vi "MergeROIs.vi"(9 "ROI 2":T1(array[cluster]), 11 "ROI 1":T1(array[cluster])) -> (3 "Merged ROI":T1(array[cluster]))   [LabVIEW 2014]
panel:
  in  "ROI":T2
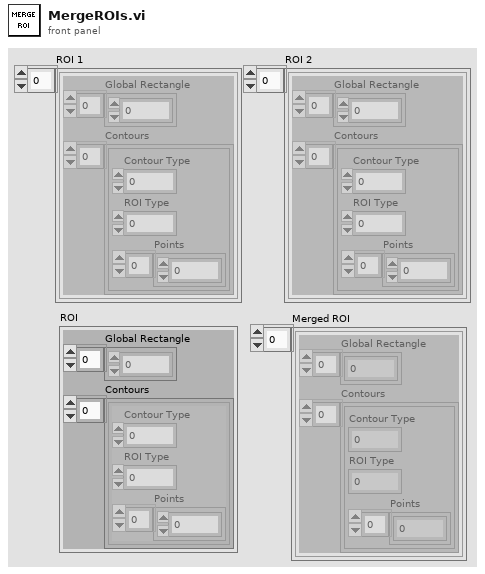
[diagram p1: front panel]
types:
  T1 = cluster{"Global Rectangle":i32[], "Contours":cluster{"Contour Type":u32, "ROI Type":u32, "Points":i32[]}[]}[]
  T2 = cluster{"Global Rectangle":i32[], "Contours":cluster{"Contour Type":u32, "ROI Type":u32, "Points":i32[]}[]}
  T3 = cluster{"Contour Type":u32, "ROI Type":u32, "Points":i32[]}[]
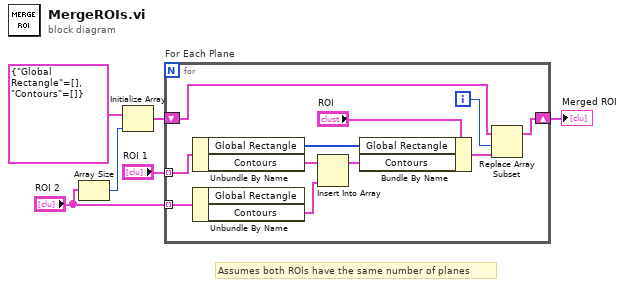
[diagram p0: block diagram]
diagram:
  # "Assumes both ROIs have the same number of planes"
  n1 = Array Size(array="ROI 2") -> (size(s)=w5:i32)
  n2 = Initialize Array(T2 {"Global Rectangle"=[], "Contours"=[]} ("ROI"), w5) -> (w3:T1)
  n3 = for "For Each Plane" {
    tunnel: "ROI 1" -> [w17] mode=indexing
    tunnel: "ROI 2" -> [w15] mode=indexing
    shift-right: [w7] -> w1
    shift-left: w3 -> [w11]
    i -> [w10]
    n4 = Unbundle By Name(w17) -> ("Global Rectangle"=w16:i32[], "Contours"=w14:T3)
    n5 = Unbundle By Name(w15) -> ("Contours"=w13:T3)  [unwired: 1 out]
    n6 = Insert Into Array(array=w14, new element=w13) -> (w12:T3)  [unwired: 1 in]
    n7 = Bundle By Name(cluster="ROI", "Global Rectangle"=w16, "Contours"=w12) -> (w8:T2)
    n8 = Replace Array Subset(array=w11, new element=w8, index=w10) -> (w7:T1)
  }
  "Merged ROI" <- w1
